vi "C37 Tester.vi"() -> ()   [LabVIEW 2013, in "C37118-DLL.lvlib"]
uses:
  C37118-DLL.lvlib
panel:
  in  "Poll Timeout [5 ms]":i32=5
  out "Difference":i32(graph)
  out "Accumulated PMU time":i32
  out "Accumulated Real Time":u32
  out "Has data? (0=no, 1=yes)":i16(graph)
  out "Pseudo PDC ID":i32
  in  "milliseconds to wait":u32
  out "Data?":bool
  out "Loop Iteration Delay":u32(graph)
  in  "stop":bool
  out "Phasor Name":string
  out "Phasor Configuration":T1
  out "PMU Configuration":T2
  out "Station Name":string
  out "pdcCfg out":T3
  out "error out":errorcluster
  in  "pdcId":i32=1001
  in  "port":i32=5011
  in  "ipAddress":string="150.106.171.173"
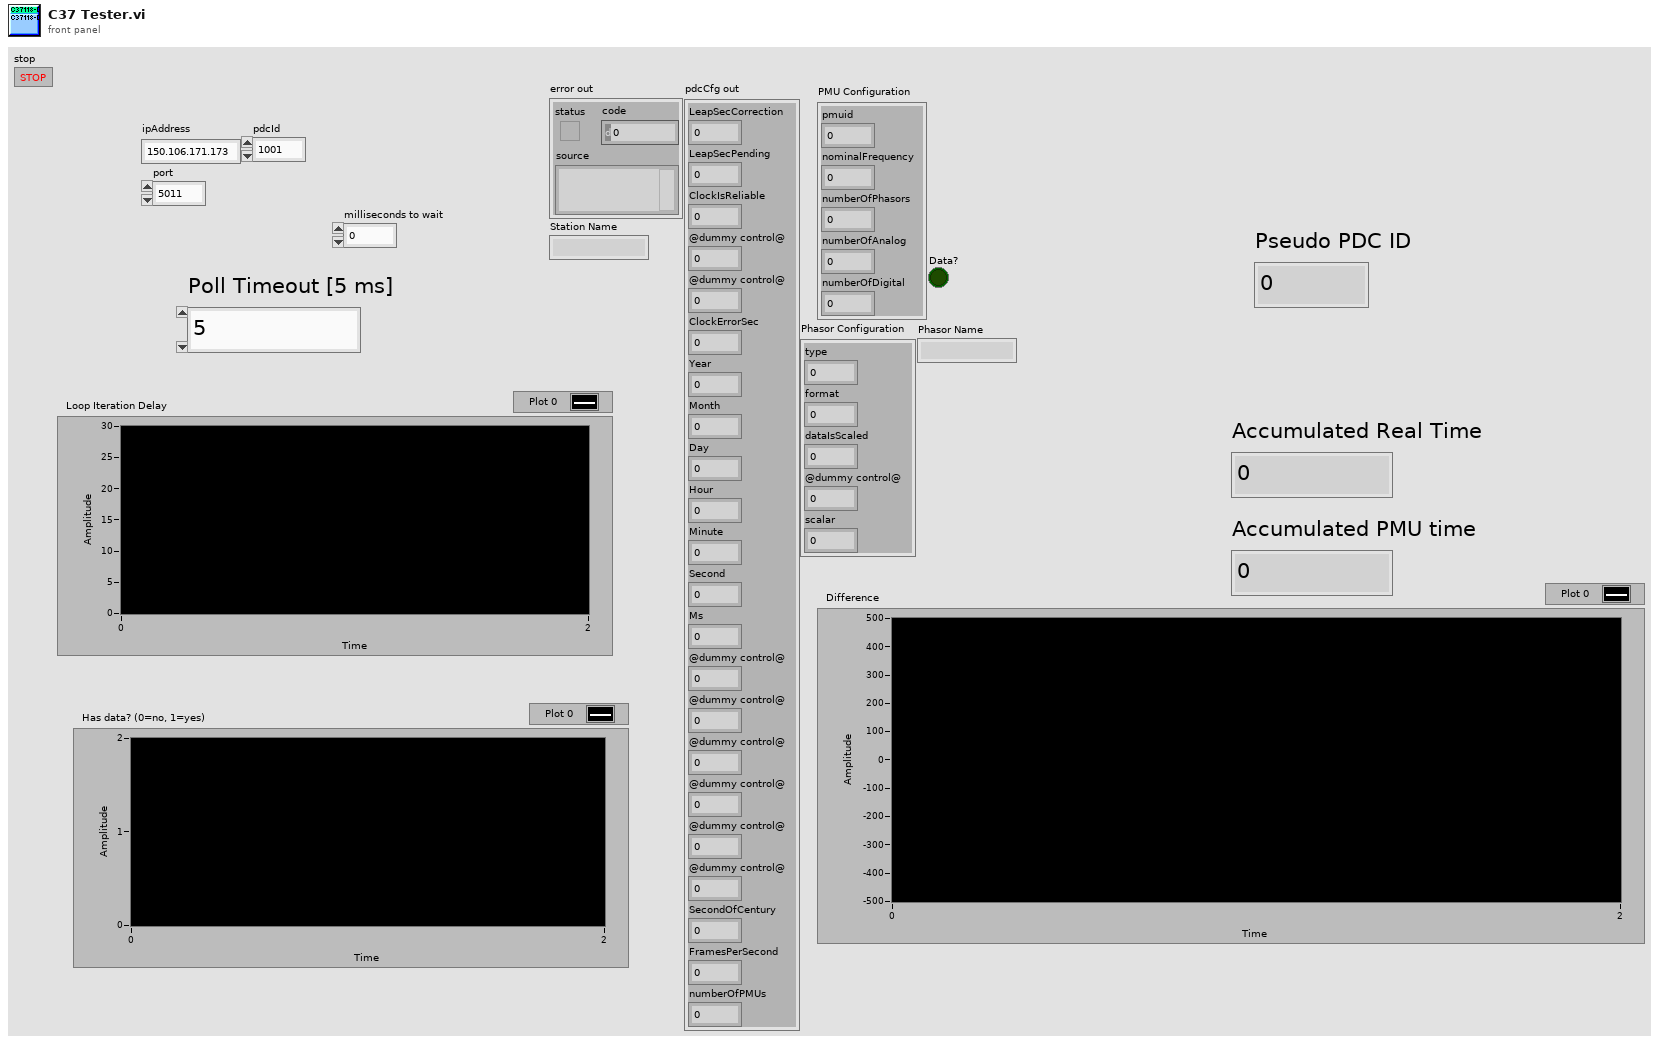
[diagram p1: front panel]
types:
  T1 = cluster{"type":u8, "format":u8, "dataIsScaled":u8, "@dummy control@":i8, "scalar":sgl}
  T2 = cluster{"pmuid":i32, "nominalFrequency":sgl, "numberOfPhasors":i32, "numberOfAnalog":i32, "numberOfDigital":i32}
  T3 = cluster{"LeapSecCorrection":i32, "LeapSecPending":u8, "ClockIsReliable":u8, "@dummy control@":i8, "@dummy control@":i8, "ClockErrorSec":sgl, "Year":i16, "Month":i16, "Day":i16, "Hour":i16, "Minute":i16, "Second":i16, "Ms":i16, "@dummy control@":i8, "@dummy control@":i8, "@dummy control@":i8, "@dummy control@":i8, "@dummy control@":i8, "@dummy control@":i8, "SecondOfCentury":dbl, "FramesPerSecond":sgl, "numberOfPMUs":i32}
  T4 = cluster{"LeapSecCorrection":i32, "LeapSecPending":u8, "ClockIsReliable":u8, "@dummy control@":i8, "@dummy control@":i8, "ClockErrorSec":sgl, "Year":i16, "Month":i16, "Day":i16, "Hour":i16, "Minute":i16, "Second":i16, "Ms":i16, "@dummy control@":i8, "@dummy control@":i8, "@dummy control@":i8, "@dummy control@":i8, "@dummy control@":i8, "@dummy control@":i8, "SecondOfCentury":dbl, "NumPmuInDataFrame":i32}
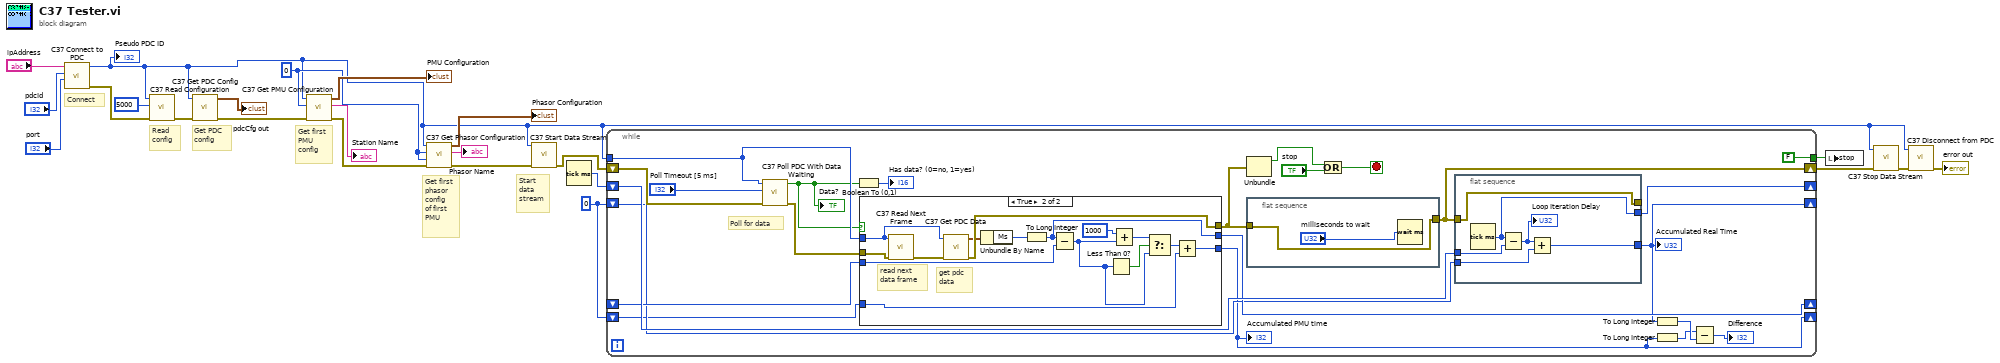
[diagram p0: block diagram]
diagram:
  w1 = i16 0 ("Ms")
  w12 = 0 ("PMU Index")
  # "Start\ndata\nstream"
  # "Get first\nphasor\nconfig \nof first\nPMU"
  # "Get first\nPMU \nconfig"
  # "Get PDC\nconfig"
  # "Read\nconfig"
  # "Connect"
  n1 = call "C37 Connect to PDC.vi"("Port"="port", "PDC ID"="pdcId", "IP Address"="ipAddress") -> ("error out"=w17:errorcluster, "Pseudo PDC ID"=w2:i32)  [unwired: 7 in]
  "Pseudo PDC ID" <- w2
  n2 = call "C37 Read Configuration.vi"("error in (no error)"=w17, "Timeout [ms]"=5000, "Pseudo PDC ID"=w2) -> ("error out"=w16:errorcluster)  [unwired: 8 in]
  n3 = call "C37 Get PDC Config.vi"("error in (no error)"=w16, "Pseudo PDC ID"=w2) -> ("error out"=w15:errorcluster, "pdcCfg out"=→"pdcCfg out":T3)  [unwired: 8 in]
  n4 = call "C37 Get PMU Configuration.vi"("error in (no error)"=w15, "PMU Index"=w12, "Pseudo PDC ID"=w2) -> ("error out"=w11:errorcluster, "Station Name"=→"Station Name":string, "PMU Configuration"=→"PMU Configuration":T2)  [unwired: 6 in]
  n5 = call "C37 Get Phasor Configuration.vi"("error in (no error)"=w11, "Phasor Index"=w12, "PMU Index"=w12, "Pseudo PDC ID"=w2) -> ("error out"=w7:errorcluster, "Channel Name"=→"Phasor Name":string, "Phasor Configuration"=→"Phasor Configuration":T1)  [unwired: 5 in]
  n6 = call "C37 Start Data Stream.vi"("error in (no error)"=w7, "Pseudo PDC ID"=w2) -> ("error out"=w6:errorcluster)  [unwired: 9 in]
  n7 = Tick Count (ms)() -> (millisecond timer value=w3:u32)
  n8 = while {
    shift-right: [w36] -> w4
    shift-left: w6 -> [w46]
    tunnel: w2 -> [w43]
    tunnel: [FALSE ("stop")] -> w8
    shift-right: [w39] -> _
    shift-left: w3 -> [w38]
    shift-right: [w33] -> _
    shift-left: _ -> [w32]
    shift-right: [w29] -> _
    shift-left: w1 -> [w31]
    shift-right: [w27] -> _
    shift-left: w1 -> [w30]
    stop <- w40 stop-if-true
    # "Poll for data"
    n9 = call "C37 Poll PDC With Data Waiting.vi"("error in (no error)"=w46, "Poll Timeout [5 ms]"="Poll Timeout [5 ms]", "Pseudo PDC ID"=w43) -> ("error out"=w44:errorcluster, "Data?"=w35:bool)  [unwired: 7 in]
    "Data?" <- w35
    n10 = Boolean To (0,1)(Boolean=w35) -> (0, 1=→"Has data? (0=no, 1=yes)":i16)
    n11 = case shown="True" w35 {
      tunnel: w44 -> [w57 w72]
      tunnel: [w57 w70] -> w37
      tunnel: w43 -> [_ w69]
      tunnel: [w55 w58] -> w33
      tunnel: w32 -> [w55 w66]
      tunnel: w30 -> [w56 w61]
      tunnel: [w56 w60] -> w27
      frame False {
      }
      frame True {
        # "get pdc\ndata"
        # "read next\ndata frame"
        n12 = call "C37 Read Next Frame.vi"("error in (no error)"=w72, "Pseudo PDC ID"=w69) -> ("error out"=w71:errorcluster)  [unwired: 9 in]
        n13 = call "C37 Get PDC Data.vi"("error in (no error)"=w71, "Pseudo PDC ID"=w69) -> ("error out"=w70:errorcluster, "PDC Data"=w68:T4)  [unwired: 8 in]
        n14 = Unbundle By Name(w68) -> ("Ms"=w67:i16)
        n15 = To Long Integer(number=w67) -> (32bit integer=w58:i32)
        n16 = Subtract(x=w58, y=w66) -> (x-y=w64:i32)
        n17 = Less Than 0?(x=w64) -> (x < 0?=w65:bool)
        n18 = Add(x=1000, y=w64) -> (x+y=w63:i32)
        n19 = Select(t=w63, s=w65, f=w64) -> (s? t:f=w59:i32)
        n20 = Add(x=w59, y=w61) -> (x+y=w60:i32)
      }
    }
    "Accumulated PMU time" <- w27
    n21 = Unbundle(w37) -> ("status"=w42:bool)  [unwired: 2 out]
    n22 = flat-sequence {
      tunnel: w37 -> [w54]
      tunnel: [w54] -> w36
      frame #0 {
        n23 = Wait (ms)(milliseconds to wait="milliseconds to wait") -> ()  [unwired: 1 out]
      }
    }
    n24 = Or(x=w42, y="stop") -> (x .or. y?=w40:bool)
    n25 = flat-sequence {
      tunnel: [w52] -> w39
      tunnel: w38 -> [w51]
      tunnel: [w50] -> _
      tunnel: w36 -> [w50]
      tunnel: w31 -> [w48]
      tunnel: [w47] -> w29
      frame #0 {
        n26 = Tick Count (ms)() -> (millisecond timer value=w52:u32)
        n27 = Subtract(x=w52, y=w51) -> (x-y=w49:u32)
        "Loop Iteration Delay" <- w49
        n28 = Add(x=w49, y=w48) -> (x+y=w47:u32)
      }
    }
    n29 = To Long Integer(number=w29) -> (32bit integer=w28:i32)
    n30 = To Long Integer(number=w27) -> (32bit integer=w26:i32)
    n31 = Subtract(x=w26, y=w28) -> (x-y=→"Difference":i32)
    "Accumulated Real Time" <- w29
  }
  n32 = local write "stop"(w8) -> ()
  n33 = call "C37 Stop Data Stream.vi"("error in (no error)"=w4, "Pseudo PDC ID"=w2) -> ("error out"=w5:errorcluster)  [unwired: 9 in]
  n34 = call "C37 Disconnect from PDC.vi"("error in (no error)"=w5, "Pseudo PDC ID"=w2) -> ("error out"=→"error out":errorcluster)  [unwired: 9 in]
